vi "Write Report Errors.vi"(8 "error in (no error)":errorcluster, 10 "Report Errors":bool, 11 "Async Message in":refnum<class "Async Message.lvclass">) -> (0 "error out":errorcluster, 3 "Async Message out":refnum<class "Async Message.lvclass">)   [LabVIEW 2023, in "Async Methods Actor.lvlib" / "Async Message.lvclass"]
doc: "If True the standard error output of the Async Method will be reported to the calling actor."
uses:
  Async Message.lvclass
  Async Message.lvclass/Async Message.ctl
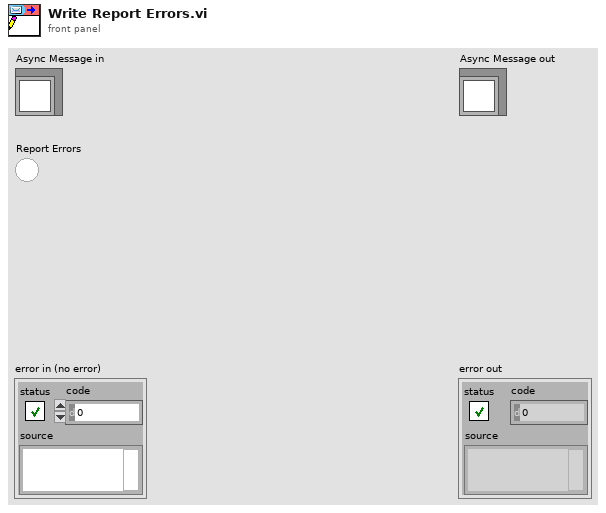
[diagram p1: front panel]
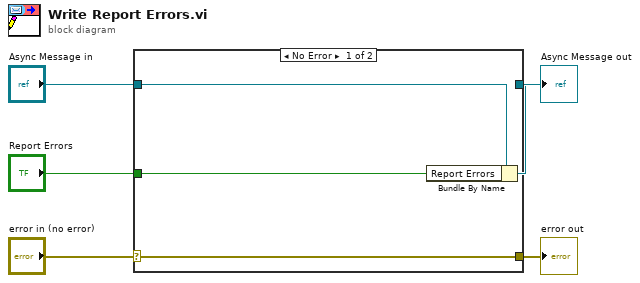
[diagram p0: block diagram]
diagram:
  n1 = case shown="No Error" "error in (no error)" {
    selector: "error in (no error)" -> [w9 w10]
    tunnel: [w9 w10] -> w4
    tunnel: [w7 w11] -> w2
    tunnel: "Async Message in" -> [w8 w11]
    tunnel: "Report Errors" -> [w6 _]
    frame No Error {
      n2 = Bundle By Name(cluster=w8, "Report Errors"=w6) -> (w7:refnum<class "Async Message.lvclass">)
    }
    frame Error {
    }
  }
  "error out" <- w4
  "Async Message out" <- w2
